vi "UWV_DAQ_V1.0.vi"() -> ()   [LabVIEW 2015]
uses:
  <vilib>/DAQmx/read.llb/DAQmx Read (Analog 2D DBL NChan NSamp).vi
  <vilib>/DAQmx/create/channels.llb/DAQmx Create Channel (AI-Voltage-Basic).vi
  <vilib>/DAQmx/configure/timing.llb/DAQmx Timing (Sample Clock).vi
  <vilib>/DAQmx/miscellaneous.llb/DAQmx Fill In Error Info.vi
panel:
  in  "save data":bool
  in  "stop":bool
  out "Waveform Graph":dbl[][](graph)
  in  "Record type":cluster{"Sampling rate":dbl, "Data":dbl[][]}
  in  "rate":dbl=1000.0 format="%0.2f"
  in  "physical channels":tag
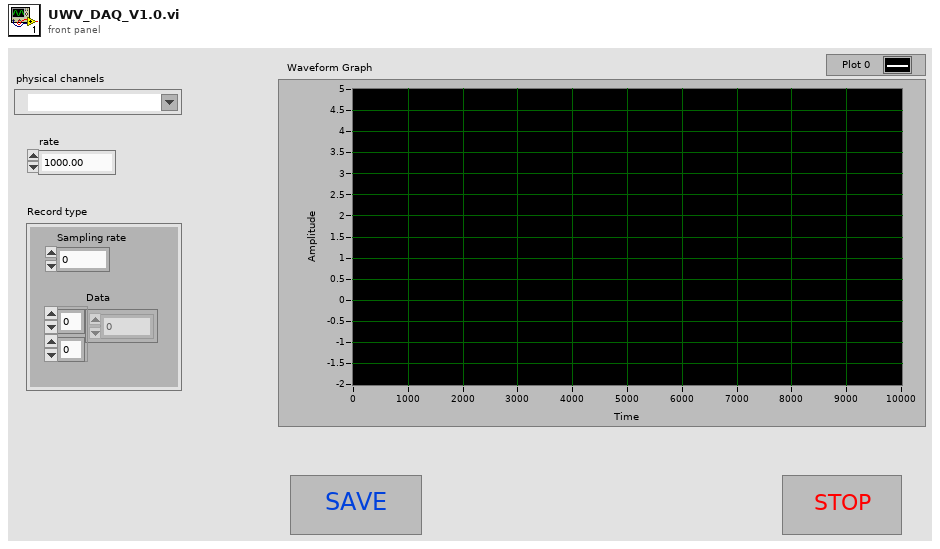
[diagram p1: front panel]
types:
  T1 = enum16{"open", "replace", "create", "open or create", "replace or create", "replace or create with confirmation"}
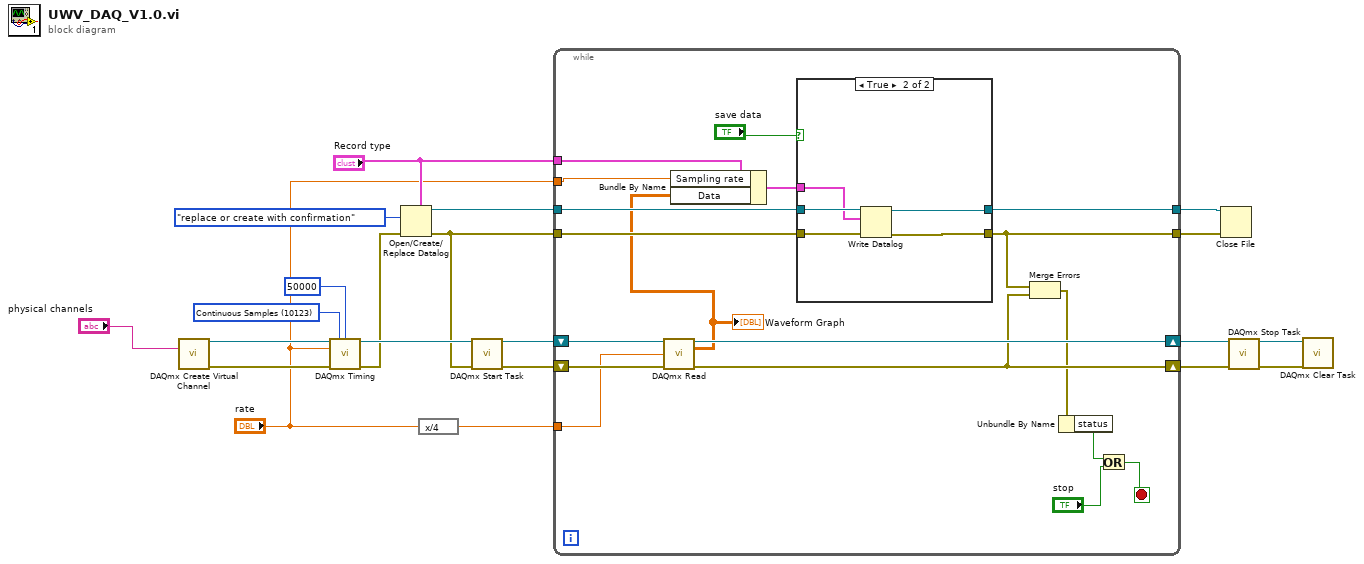
[diagram p0: block diagram]
diagram:
  w13 = 10123 items=["Finite Samples"=10178, "Continuous Samples"=10123, "Hardware Timed Single Point"=12522] ("sample mode")
  n1 = call-poly <vilib>:"DAQmx Create Virtual Channel.vi"("physical channels"="physical channels") -> ("task out"=w21:refnum<k21>, "error out"=w17:errorcluster)  [unwired: 13 in]
  n2 = call-poly <vilib>:"DAQmx Timing.vi"("task/channels in"=w21, "sample mode"=w13, "samples per channel"=50000, "rate"="rate", "error in"=w17) -> ("task out"=w20:refnum<k21>, "error out"=w8:errorcluster)  [unwired: 9 in]
  n3 = Open/Create/Replace Datalog(5:"Record type", 8:w8, 10:T1."replace or create with confirmation" ("operation (0:open)")) -> (0:w7:errorcluster, 3:w9:refnum<k1>)  [unwired: 3 in, 1 out]
  n4 = expression code="x/4"("rate") -> (w6:dbl)
  n5 = call <vilib>:"DAQmx Start Task.vi"("task/channels in"=w20, "error in"=w7) -> ("task out"=w19:refnum<k21>, "error out"=w16:errorcluster)  [unwired: 12 in]
  n6 = while {
    shift-right: [w38] -> w18
    shift-left: w19 -> [w39]
    shift-right: [w27] -> w15
    shift-left: w16 -> [w37]
    tunnel: w9 -> [w35]
    tunnel: w7 -> [w34]
    tunnel: w6 -> [w36]
    tunnel: "Record type" -> [w33]
    tunnel: "rate" -> [w32]
    tunnel: [w28] -> w3
    tunnel: [w29] -> w2
    stop <- w25 stop-if-true
    n7 = call-poly <vilib>:"DAQmx Read.vi"("task/channels in"=w39, "number of samples per channel"=w36, "error in"=w37) -> ("task out"=w38:refnum<k21>, "data"=w31:dbl[][], "error out"=w27:errorcluster)  [unwired: 10 in]
    "Waveform Graph" <- w31
    n8 = Bundle By Name(cluster=w33, "Sampling rate"=w32, "Data"=w31) -> (w30:cluster{"Sampling rate":dbl, "Data":dbl[][]})
    n9 = case shown="True" "save data" {
      tunnel: w35 -> [w41 w45]
      tunnel: w34 -> [w40 w46]
      tunnel: [w41 w44] -> w29
      tunnel: [w40 w43] -> w28
      tunnel: w30 -> [_ w42]
      frame False {
      }
      frame True {
        n10 = Write Datalog(4:w46, 6:w42, 7:w45) -> (0:w43:errorcluster, 3:w44:refnum<k1>)
      }
    }
    n11 = Merge Errors(w28, w27) -> (w26:errorcluster)
    n12 = Unbundle By Name(w26) -> ("status"=w24:bool)
    n13 = Or(x=w24, y="stop") -> (x .or. y?=w25:bool)
  }
  n14 = Close File(refnum=w2, error in=w3) -> ()  [unwired: 2 out]
  n15 = call <vilib>:"DAQmx Stop Task.vi"("task/channels in"=w18, "error in"=w15) -> ("task out"=w11:refnum<k21>, "error out"=w10:errorcluster)  [unwired: 12 in]
  n16 = call <vilib>:"DAQmx Clear Task.vi"("task in"=w11, "error in"=w10) -> ()  [unwired: 13 in, 1 out]
